vi "Main GUI.vi"() -> ()   [LabVIEW 2014]
uses:
  Hardware/Translation Stage/Ctrls/Motion Translation Module Control.ctl
  C:/Projects/Serial Sectioning OCT/Software/Thorlabs.MotionControl.IntegratedStepperMotorsCLI.dll
  Thorlabs.MotionControl.IntegratedStepperMotorsCLI.dll
  C:/Projects/Serial Sectioning OCT/Software/Thorlabs.MotionControl.Controls.dll
  Thorlabs.MotionControl.Controls.dll
panel:
  in  "LongTravelStageControl":refnum<k24>(container)
  in  "Uninit Motor":bool
  in  "Init Motor":bool
  in  "Stop Button":bool
  in  "Y Axis":T1={"Device"=refnum, "Device SN"="45876060", "Is.Connected?"=TRUE, "Is.Enabled?"=TRUE, "DevicePosition"=0.0}
  out "Error Out":errorcluster={"status"=TRUE, "code"=1172, "source"="Property Node (Arg :1) Error accessing property Thorlabs.MotionControl.Controls.LongTravelStageControl.IsConnected, (System.ArgumentNullException: Key cannot be null.\r\nParameter name: key) <append><b>System.ArgumentNullException</b> in Motion Control Module.vi:2250001->Main GUI.vi"}
  in  "X Axis":T1={"Device"=refnum, "Device SN"="45876539", "Is.Connected?"=TRUE, "Is.Enabled?"=TRUE, "DevicePosition"=0.0}
  in  "X Axis":refnum<k24>(container)
  in  "Error In":errorcluster
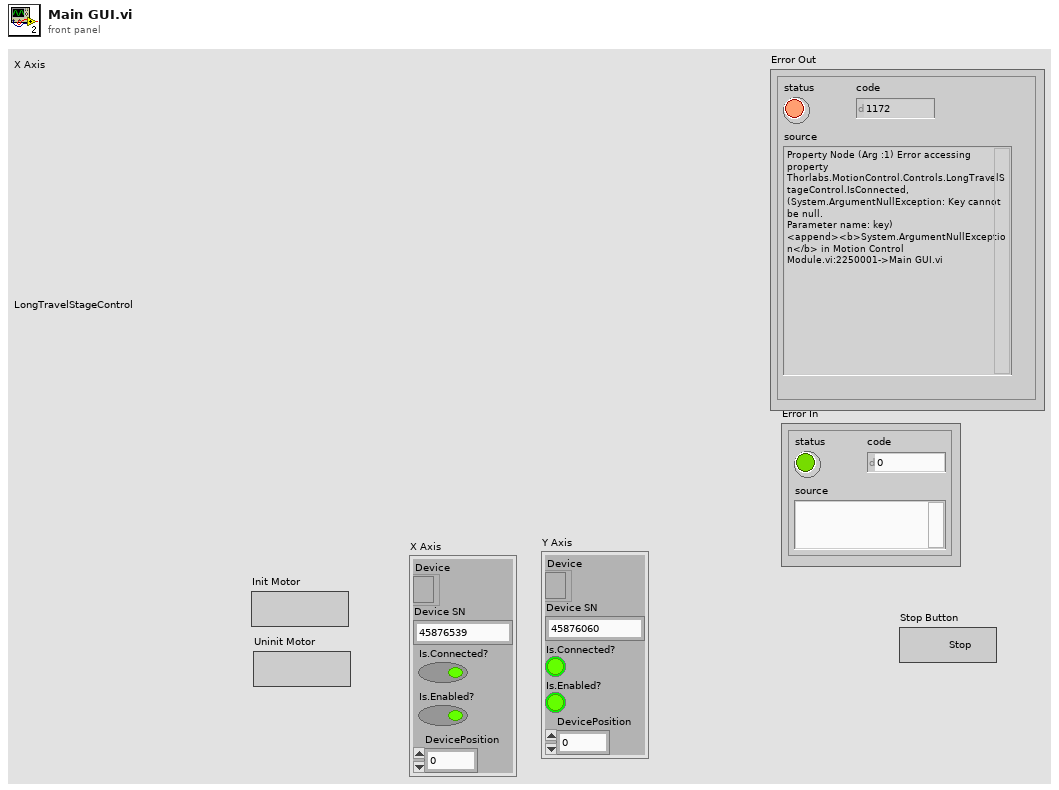
[diagram p1: front panel]
types:
  T1 = cluster{"Device":refnum<k24>, "Device SN":string, "Is.Connected?":bool, "Is.Enabled?":bool, "DevicePosition":dbl}
  T2 = typedef "Motion Translation Module Control.ctl" = enum16{"Init", "Home", "Configure", "Position", "Jog", "Stop", "Uninit"}
  T3 = typedef "Translation Stage Cluster.ctl" = cluster{"Device SN":string, "Is.Connected?":bool, "Is.Enabled?":bool, "Position":dbl, "AccelerationMaximum":dbl, "VelocityMaximum":dbl, "Acceleration":dbl, "Velocity":dbl, "waitTimeout (ms)":i32}
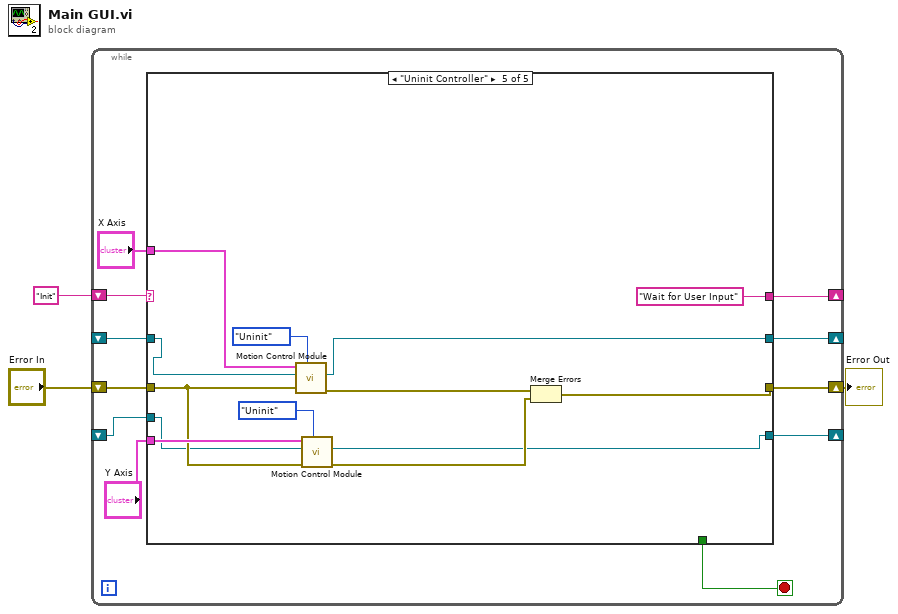
[diagram p0: block diagram]
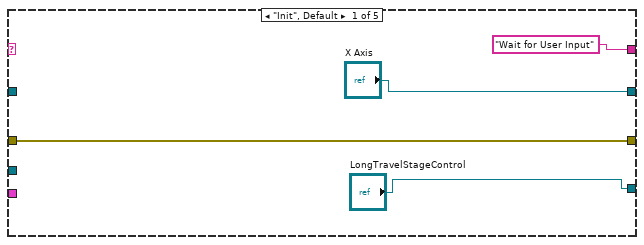
[diagram p2: hidden frame]
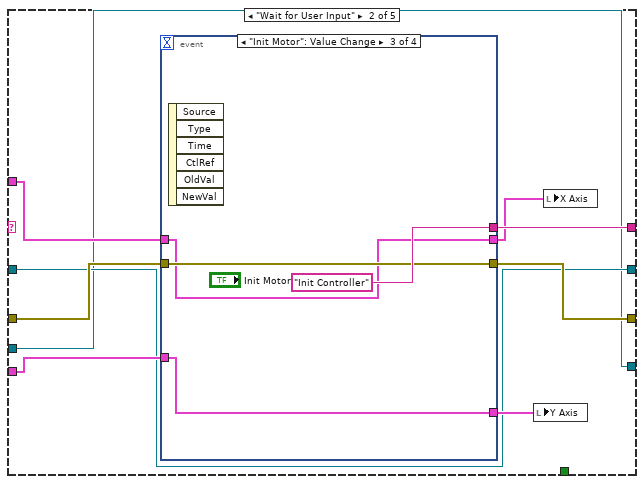
[diagram p3: hidden frame]
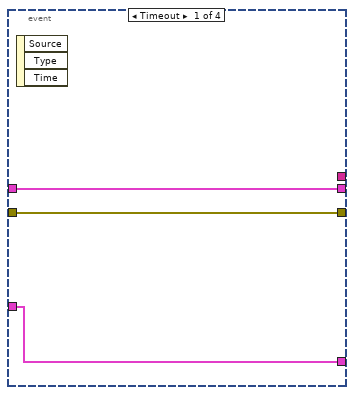
[diagram p4: hidden frame]
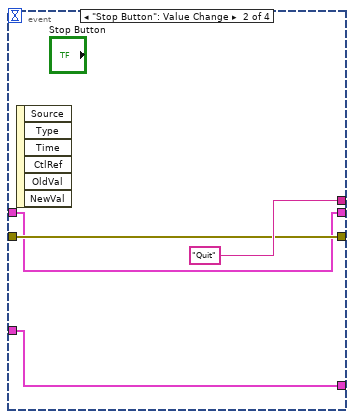
[diagram p5: hidden frame]
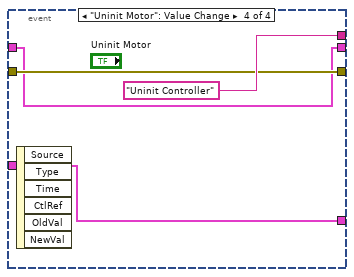
[diagram p6: hidden frame]
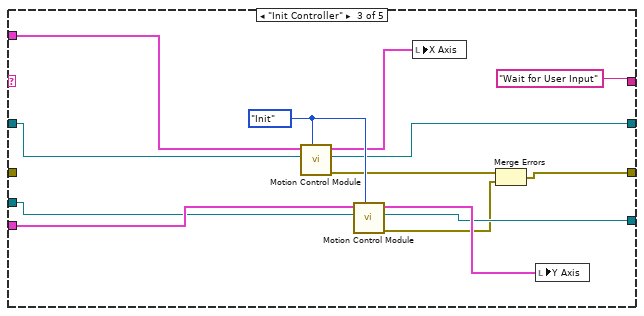
[diagram p7: hidden frame]
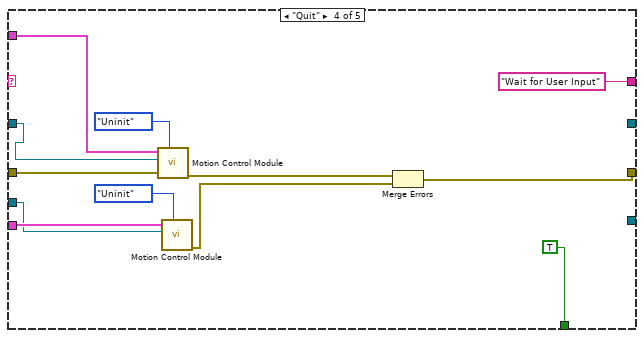
[diagram p8: hidden frame]
diagram:
  n1 = while {
    shift-right: [w12] -> _
    shift-left: "Init" -> [w13]
    shift-right: [w10] -> w1
    shift-left: "Error In" -> [w11]
    shift-right: [w7] -> _
    shift-left: _ -> [w6]
    shift-right: [w5] -> _
    shift-left: _ -> [w4]
    stop <- w14 stop-if-true
    n2 = case shown="\"Uninit Controller\"" w13 {
      tunnel: [_ _ _ TRUE _] -> w14
      tunnel: ["Wait for User Input" w27 "Wait for User Input" "Wait for User Input" "Wait for User Input"] -> w12
      tunnel: w11 -> [w17 w26 _ w65 w74]
      tunnel: [w17 w25 w45 w57 w73] -> w10
      tunnel: "X Axis" -> [_ w24 w54 w60 w77]
      tunnel: "Y Axis" -> [_ w22 w53 w61 w75]
      tunnel: ["LongTravelStageControl" w19 w49 _ w68] -> w7
      tunnel: w6 -> [_ w19 w43 w58 w71]
      tunnel: ["X Axis" w20 w48 _ w69] -> w5
      tunnel: w4 -> [_ w20 w44 w59 w70]
      frame "Init", Default {
      }
      frame "Wait for User Input" {
        n3 = event shown="[2] \"Init Motor\": Value Change" {
          selector: _ -> [_ _ _ _]
          dyn-events: _ -> [_ _ _ _]
          timeout: _ -> [_ _ _ _]
          tunnel: [_ "Quit" "Init Controller" "Uninit Controller"] -> w27
          tunnel: w26 -> [w28 w33 w37 w41]
          tunnel: [w28 w33 w37 w41] -> w25
          tunnel: w24 -> [w29 w32 w36 w40]
          tunnel: [w29 w32 w36 w40] -> w23
          tunnel: w22 -> [w30 w31 w35 w39]
          tunnel: [w30 w31 w35 w39] -> w21
          event Timeout {
            n4 = event-data() -> ()  [unwired: 1 in, 3 out]
          }
          event "Stop Button": Value Change {
            n5 = event-data() -> ()  [unwired: 1 in, 6 out]
          }
          event "Init Motor": Value Change {
            n6 = event-data() -> ()  [unwired: 1 in, 6 out]
          }
          event "Uninit Motor": Value Change {
            n7 = event-data() -> ()  [unwired: 1 in, 6 out]
          }
        }
        n8 = local write "Y Axis"(w21) -> ()
        n9 = local write "X Axis"(w23) -> ()
      }
      frame "Init Controller" {
        w52 = Motion_Translation_Module_Control."Init"
        n10 = call "Motion Control Module.vi"("Action"=w52, "LTS Reference"=w44, "Cluster"=w54) -> ("Error Out"=w47:errorcluster, "LTS Reference Out"=w48:refnum<k24>, "Cluster"=w51:T3)  [unwired: 6 in]
        n11 = call "Motion Control Module.vi"("Action"=w52, "LTS Reference"=w43, "Cluster"=w53) -> ("Error Out"=w46:errorcluster, "LTS Reference Out"=w49:refnum<k24>, "Cluster"=w50:T3)  [unwired: 6 in]
        n12 = local write "X Axis"(w51) -> ()
        n13 = Merge Errors(w47, w46) -> (w45:errorcluster)
        n14 = local write "Y Axis"(w50) -> ()
      }
      frame "Quit" {
        n15 = call "Motion Control Module.vi"("Action"=Motion_Translation_Module_Control."Uninit", "Error In"=w65, "LTS Reference"=w59, "Cluster"=w60) -> ("Error Out"=w64:errorcluster)  [unwired: 5 in, 2 out]
        n16 = call "Motion Control Module.vi"("Action"=Motion_Translation_Module_Control."Uninit", "LTS Reference"=w58, "Cluster"=w61) -> ("Error Out"=w56:errorcluster)  [unwired: 6 in, 2 out]
        n17 = Merge Errors(w64, w56) -> (w57:errorcluster)
      }
      frame "Uninit Controller" {
        n18 = call "Motion Control Module.vi"("Action"=Motion_Translation_Module_Control."Uninit", "Error In"=w74, "LTS Reference"=w70, "Cluster"=w77) -> ("Error Out"=w79:errorcluster, "LTS Reference Out"=w69:refnum<k24>)  [unwired: 5 in, 1 out]
        n19 = call "Motion Control Module.vi"("Action"=Motion_Translation_Module_Control."Uninit", "Error In"=w74, "LTS Reference"=w71, "Cluster"=w75) -> ("Error Out"=w72:errorcluster, "LTS Reference Out"=w68:refnum<k24>)  [unwired: 5 in, 1 out]
        n20 = Merge Errors(w79, w72) -> (w73:errorcluster)
      }
    }
  }
  "Error Out" <- w1
